vi "Read test Data.vi"() -> ()   [LabVIEW 2011]
uses:
  e:/NI Temp/Clemessy RM 2013 13/RefMem DMA/Source/Custom Device/Real-Time/SubVIs/Block descriptor.ctl
  e:/NI Temp/Clemessy RM 2013 13/RefMem DMA/Source/Custom Device/RefMem DMA Custom Device.lvlib
panel:
  out "read":T1[](array[typedef])
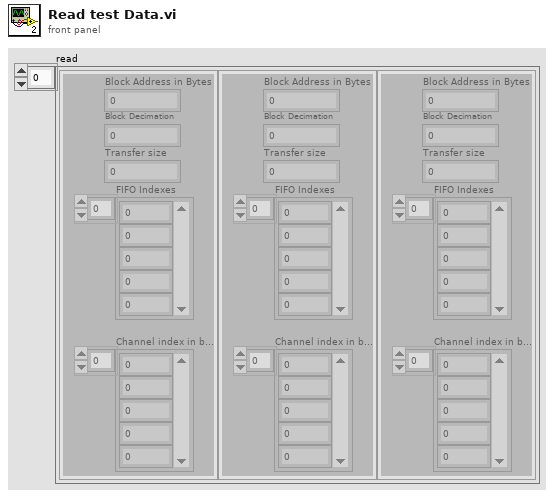
[diagram p1: front panel]
types:
  T1 = typedef "RefMem DMA Custom Device.lvlib/Block descriptor.ctl" = cluster{"Block Address in Bytes":u32, "Block Decimation":u32, "Transfer size":u32, "FIFO Indexes":i32[], "Channel index in block":i32[]}
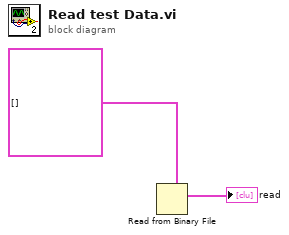
[diagram p0: block diagram]
diagram:
  n1 = Read from Binary File(5:T1[] [] ("Read Block Descriptors")) -> (2:→"read":T1[])  [unwired: 5 in, 3 out]
